vi "SOUR_POW_CORR_COLL_C_SEN_FRAN.vi"(0 "VISA IN":refnum<visa-resource-name>, 1 "Power Meter Channel":string, 2 "Min Frq.":i32, 3 "Max Frq.":i32, 5 "error in":errorcluster, 7 "Channel":i32) -> (14 "VISA Out":refnum<visa-resource-name>, 19 "error out":errorcluster)   [LabVIEW 2018, in "PNA-X.lvlib"]
doc: "SOURce<cnum>:POWer:CORRection:COLLect:<pmChan>SENsor[:FRANge] \n<num1>,<num2> \n1841\n\n(Read-Write) Specifies the frequency range over which the power sensors connected to the specified \nchannels (A and B) of the power meter can be used (minimum frequency, maximum frequency). If the \npower meter has only a single channel, that channel is considered channel A. \nParameters \n<cnum> Any existing channel number. If unspecified, value is set to 1 \n<pmChan> Power Meter channel. Choose from: \nA - Channel A \nB - Channel B \n<num1> Minimum frequency for the sensor. If a frequency unit is not specified, Hz is \nassumed. No limits are placed on this value. \n<num2> Maximum frequency for the sensor. If a frequency unit is not specified, Hz is \nassumed. No limits are placed on this value. \nExamples SOUR:POW:CORR:COLL:ASEN 100E3, 3E9 \nsource1:power2:correction:collect:bsensor:frange 10 MHz, 18 GHz \nQuery Syntax SOURce:POWer:CORRection:COLLect:ASENsor[:FRANge]? \nSOURce:POWer:CORRection:COLLect:BSENsor[:FRANge]? \nReturn Type Numeric \nDefault 0,0"
uses:
  PNA-X.lvlib
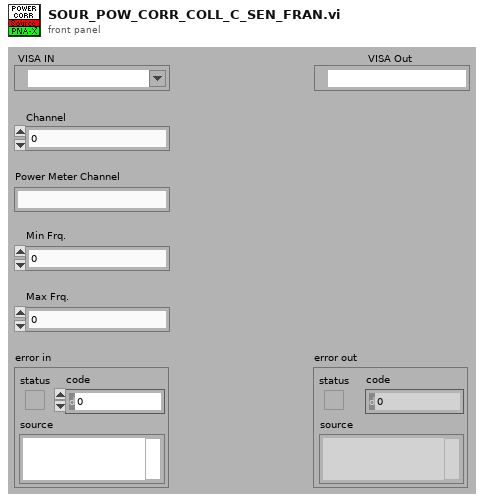
[diagram p1: front panel]
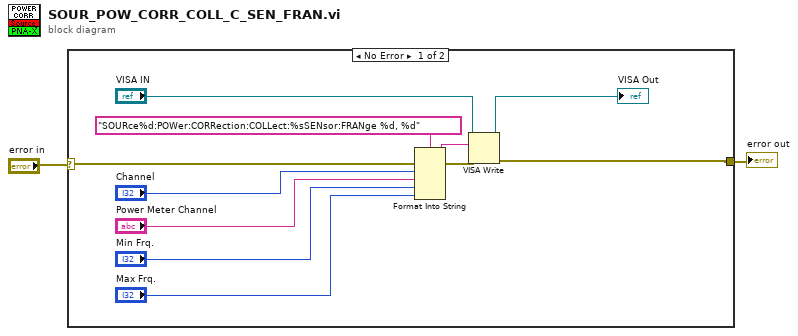
[diagram p0: block diagram]
diagram:
  n1 = case shown="No Error" "error in" {
    selector: "error in" -> [w13 w14]
    tunnel: [w8 w14] -> w1
    frame No Error {
      n2 = Format Into String(format string="SOURce%d:POWer:CORRection:COLLect:%sSENsor:FRANge %d, %d" ("Cmdline"), error in=w13, "Channel", "Power Meter Channel", "Min Frq.", "Max Frq.") -> (resulting string=w11:string, error out=w12:errorcluster)  [unwired: 1 in]
      n3 = VISA Write(VISA resource name="VISA IN", write buffer=w11, error in (no error)=w12) -> (VISA resource name out=→"VISA Out":refnum<visa-resource-name>, error out=w8:errorcluster)  [unwired: 1 out]
    }
    frame Error {
    }
  }
  "error out" <- w1
